vi "test_libssh2_session_hostkey.vi"() -> ()   [LabVIEW 2017, in "integration_tests.lvlib"]
uses:
  integration_tests.lvlib
  libssh2/libssh2_session_handshake_tcp.vi
  libssh2/libssh2_init_default.vi
  libssh2/libssh2_session_init_ex.vi
  <vilib>/Utility/tcp.llb/TCP Get Raw Net Object.vi
  libssh2/libssh2_session_handshake_socket.vi
  libssh2/libssh2.lvlib
  support/support.lvlib
  <vilib>/PNR/Transparent Assertions/Transparent Assertions/Transparent Assertions.lvlib
panel:
  out "error out":errorcluster
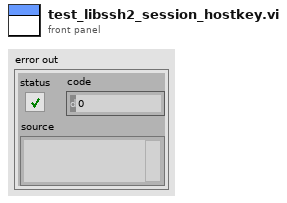
[diagram p1: front panel]
types:
  T1 = typedef "libssh2.lvlib/Session Refnum.ctl" = refnum<k1>
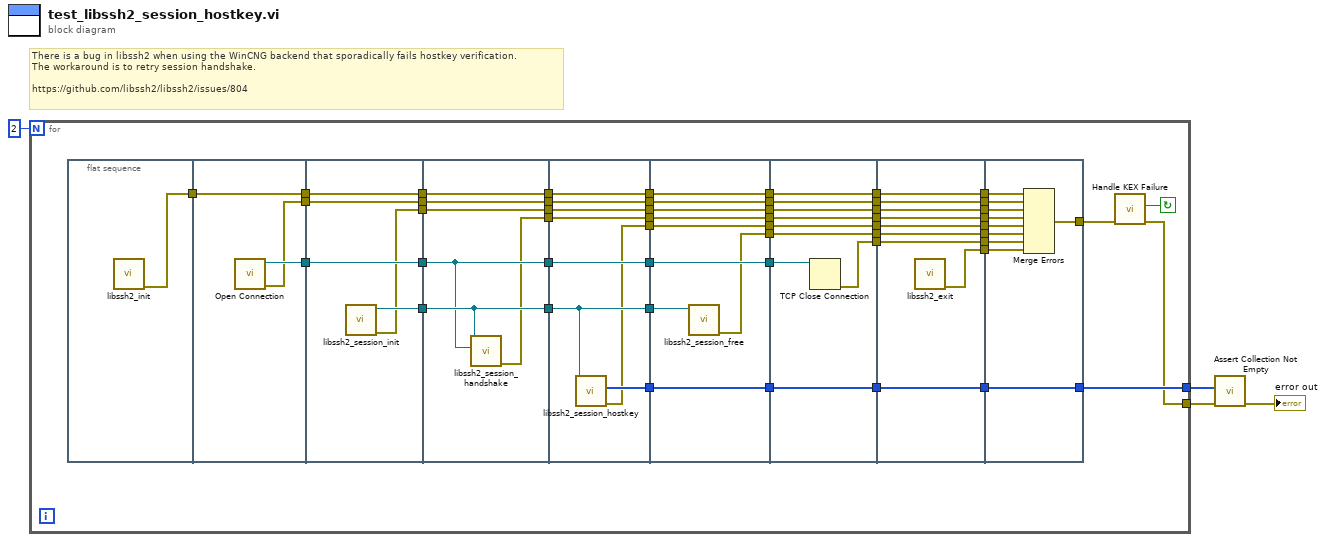
[diagram p0: block diagram]
diagram:
  # "There is a bug in libssh2 when using the WinCNG backend that sporadically fails hostkey verification.\nThe workaround is to retry session handshake.\n\nhttps://github.com/libssh2/libssh2/issues/804"
  n1 = for {
    N: 2 -> [_]
    tunnel: [w8] -> w3
    tunnel: [w5] -> w1
    stop <- w6 continue-if-true
    n2 = flat-sequence {
      tunnel: [w57] -> w56
      tunnel: [w60] -> w55
      tunnel: w56 -> [w59]
      tunnel: [w59] -> w54
      tunnel: [w58] -> w53
      tunnel: w55 -> [w65]
      tunnel: [w65] -> w52
      tunnel: w54 -> [w64]
      tunnel: [w64] -> w51
      tunnel: w53 -> [w63]
      tunnel: [w63] -> w50
      tunnel: [w62] -> w49
      tunnel: [w61] -> w48
      tunnel: w52 -> [w67]
      tunnel: [w67] -> w47
      tunnel: w51 -> [w71]
      tunnel: [w71] -> w46
      tunnel: w50 -> [w70]
      tunnel: [w70] -> w45
      tunnel: [w69] -> w44
      tunnel: w49 -> [w69]
      tunnel: w48 -> [w68]
      tunnel: [w68] -> w43
      tunnel: [w66] -> w42
      tunnel: w47 -> [w79]
      tunnel: [w79] -> w41
      tunnel: w46 -> [w78]
      tunnel: [w78] -> w40
      tunnel: w45 -> [w77]
      tunnel: [w77] -> w39
      tunnel: w44 -> [w73]
      tunnel: [w73] -> w38
      tunnel: w43 -> [w76]
      tunnel: [w76] -> w37
      tunnel: [w74] -> w36
      tunnel: w42 -> [w75]
      tunnel: [w75] -> w35
      tunnel: [w72] -> w34
      tunnel: w41 -> [w88]
      tunnel: [w88] -> w33
      tunnel: w40 -> [w87]
      tunnel: [w87] -> w32
      tunnel: w39 -> [w86]
      tunnel: [w86] -> w31
      tunnel: w38 -> [w85]
      tunnel: w37 -> [w84]
      tunnel: [w84] -> w30
      tunnel: [w83] -> w29
      tunnel: w36 -> [w82]
      tunnel: [w82] -> w28
      tunnel: w35 -> [w81]
      tunnel: [w81] -> w27
      tunnel: w34 -> [w80]
      tunnel: [w80] -> w26
      tunnel: w33 -> [w97]
      tunnel: w32 -> [w96]
      tunnel: [w96] -> w25
      tunnel: w31 -> [w95]
      tunnel: [w95] -> w24
      tunnel: [w94] -> w23
      tunnel: w30 -> [w93]
      tunnel: [w93] -> w22
      tunnel: w29 -> [w92]
      tunnel: [w92] -> w21
      tunnel: w28 -> [w91]
      tunnel: [w91] -> w20
      tunnel: w27 -> [w90]
      tunnel: [w90] -> w19
      tunnel: w26 -> [w89]
      tunnel: [w89] -> w18
      tunnel: w25 -> [w106]
      tunnel: [w106] -> w17
      tunnel: w24 -> [w105]
      tunnel: [w105] -> w16
      tunnel: w23 -> [w104]
      tunnel: [w104] -> w15
      tunnel: [w103] -> w14
      tunnel: w22 -> [w102]
      tunnel: [w102] -> w13
      tunnel: w21 -> [w101]
      tunnel: [w101] -> w12
      tunnel: w20 -> [w100]
      tunnel: [w100] -> w11
      tunnel: w19 -> [w99]
      tunnel: [w99] -> w10
      tunnel: w18 -> [w98]
      tunnel: [w98] -> w9
      tunnel: w17 -> [w116]
      tunnel: w16 -> [w115]
      tunnel: w15 -> [w114]
      tunnel: w14 -> [w113]
      tunnel: w13 -> [w112]
      tunnel: w12 -> [w111]
      tunnel: w11 -> [w108]
      tunnel: w10 -> [w110]
      tunnel: w9 -> [w109]
      tunnel: [w108] -> w8
      tunnel: [w107] -> w7
      frame #0 {
        n3 = call-poly "libssh2_init.vi"() -> ("error out"=w57:errorcluster)  [unwired: 11 in]
      }
      frame #1 {
        n4 = call "Open Connection.vi"() -> ("error out"=w58:errorcluster, "connection ID"=w60:refnum<k5>)  [unwired: 10 in]
      }
      frame #2 {
        n5 = call "libssh2_session_init.vi"() -> ("error out"=w61:errorcluster, "session"=w62:T1)  [unwired: 10 in]
      }
      frame #3 {
        n6 = call-poly "libssh2_session_handshake.vi"("tcp connection"=w67, "session"=w69) -> ("error out"=w66:errorcluster)  [unwired: 9 in]
      }
      frame #4 {
        n7 = call "libssh2_session_hostkey.vi"("session"=w73) -> ("error out"=w72:errorcluster, "hostkey"=w74:u8[])  [unwired: 8 in, 1 out]
      }
      frame #5 {
        n8 = call "libssh2_session_free.vi"("session"=w85) -> ("error out"=w83:errorcluster)  [unwired: 10 in]
      }
      frame #6 {
        n9 = TCP Close Connection(connection ID=w97) -> (error out=w94:errorcluster)  [unwired: 2 in, 1 out]
      }
      frame #7 {
        n10 = call "libssh2_exit.vi"() -> ("error out"=w103:errorcluster)  [unwired: 11 in]
      }
      frame #8 {
        n11 = Merge Errors(w116, w115, w112, w110, w109, w111, w114, w113) -> (w107:errorcluster)
      }
    }
    n12 = call "Handle KEX Failure.vi"("error in (no error)"=w7) -> ("error out"=w5:errorcluster, "KEX Failure"=w6:bool)  [unwired: 9 in]
  }
  n13 = call <vilib>:"Assert Collection Not Empty.vi"("error in (no error)"=w1, "Collection"=w3) -> ("error out"=→"error out":errorcluster)  [unwired: 9 in]
